vi "Search Tree Path.vi"(8 "Error In":errorcluster, 10 "Tree Path":string, 11 "Tree Manager":T1) -> (0 "Error Out":errorcluster, 1 "Tree ID":string, 3 "Tree Manager":T1)   [LabVIEW 2016, in "Tree Manager.lvclass"]
doc: "Search by using the specified Tree Path. The Tree Path should contain a sequence of names, each index specifying another level. The syntax should mimic a web URL with / symbols between levels.\n\nExample: Parent/Nested1/Nested2/Nested3 corresponds to a Tree with 4 levels, each containing one Child Tree."
uses:
  Tree Manager.lvclass
  Typedefs/Session Handle.ctl
  <vilib>/Utility/error.llb/Error Cluster From Error Code.vi
  <vilib>/ErrorRing/Error Ring.xnode
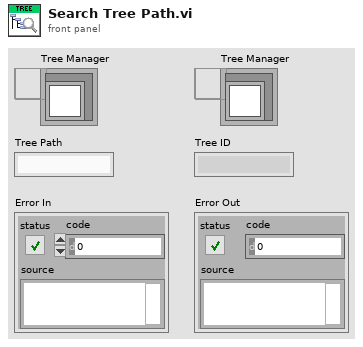
[diagram p1: front panel]
types:
  T1 = typedef "Tree Manager.lvclass/Session Handle.ctl" = refnum<data-value>
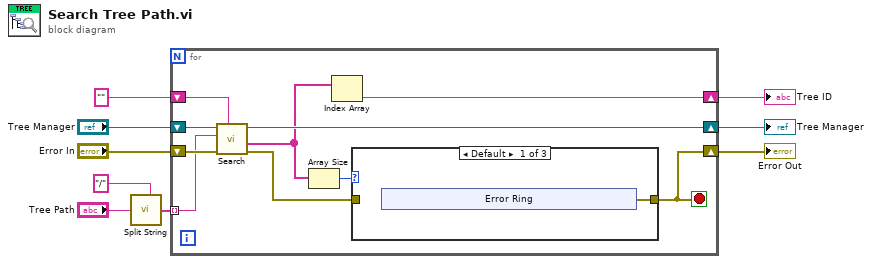
[diagram p0: block diagram]
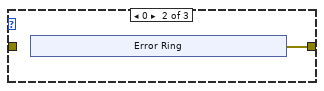
[diagram p2: hidden frame]
diagram:
  n1 = call <vilib>:"Split String.vi"("Split Pattern"="/", "Input String"="Tree Path") -> ("Split String"=w1:string[])  [unwired: 5 in]
  n2 = for {
    shift-right: [w18] -> w7
    shift-left: "Tree Manager" -> [w19]
    tunnel: w1 -> [w10] mode=indexing
    shift-right: [w17] -> w9
    shift-left: "" ("Unique ID") -> [w11]
    shift-right: [w13] -> w8
    shift-left: "Error In" -> [w16]
    stop <- w13 stop-if-true
    n3 = call "Search.vi"("Parent ID"=w11, "Error In"=w16, "Name"=w10, "Tree Manager"=w19) -> ("Error Out"=w14:errorcluster, "IDs"=w12:string[], "Tree Manager"=w18:T1)  [unwired: 5 in]
    n4 = Array Size(array=w12) -> (size(s)=w15:i32)
    n5 = Index Array(array=w12) -> (element=w17:string)  [unwired: 1 in]
    n6 = case shown="Default" w15 {
      tunnel: w14 -> [_ _ w32]
      tunnel: [w20 w26 w32] -> w13
      frame Default {
        n7 = xnode "Error Ring"() -> ("error out"=w20:errorcluster)
      }
      frame 0 {
        n8 = xnode "Error Ring"() -> ("error out"=w26:errorcluster)
      }
      frame 1 {
      }
    }
  }
  "Tree ID" <- w9
  "Error Out" <- w8
  "Tree Manager" <- w7
